vi "mqttInterpretSubscribtionData.vi"(0 "rxTelegram in":u8[](array[numeric]) format="%02x", 5 "qos":T1, 11 "error in (no error)":errorcluster) -> (4 "topic":string, 6 "value":string, 8 "messageID":u16, 15 "error out":errorcluster)   [LabVIEW 2015, in "mqtt.lvclass"]
uses:
  mqtt.lvclass
  mqttTypedef/mqttQOSlevel.ctl
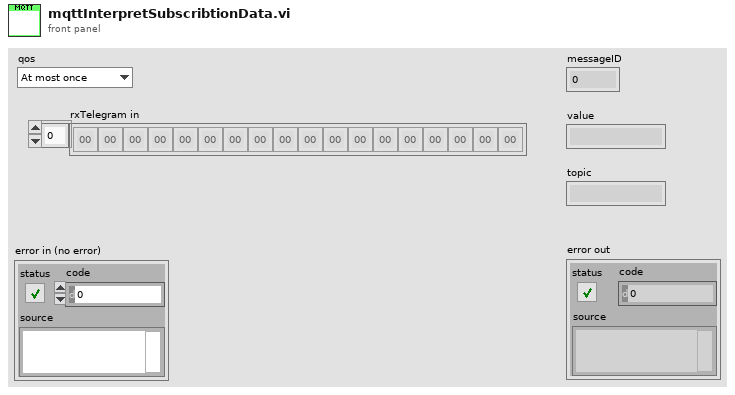
[diagram p1: front panel]
types:
  T1 = typedef "mqttQOSlevel.ctl" = enum8{"At most once", "At least once", "Exactly once", "Reserved"}
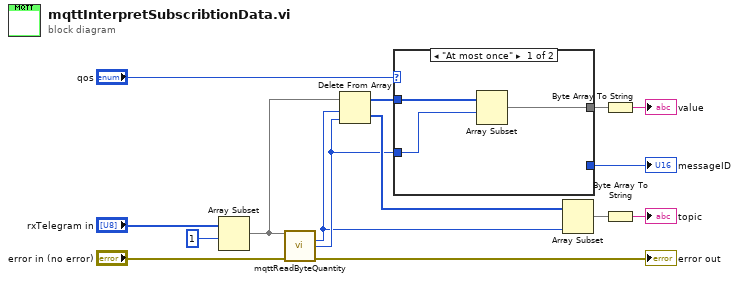
[diagram p0: block diagram]
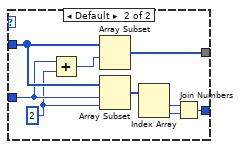
[diagram p2: hidden frame]
diagram:
  n1 = Array Subset(array="rxTelegram in", index=1) -> (w6:u8[])  [unwired: 1 in]
  n2 = call "mqttReadByteQuantity.vi"("rxTelegram in"=w6, "error in (no error)"="error in (no error)") -> ("remainingLength"=w1:i32, "lengthByteQuantity"=w2:i32, "error out"=→"error out":errorcluster)  [unwired: 11 in]
  n3 = Delete From Array(array=w6, length=w1, index=w2) -> (deleted portion=w4:u8[], array with subset deleted=w3:u8[])
  n4 = case shown="\"At most once\"" "qos" {
    tunnel: w3 -> [w18 w22]
    tunnel: [_ w25] -> w12
    tunnel: [w17 w23] -> w5
    tunnel: w2 -> [w16 w21]
    frame "At most once" {
      n5 = Array Subset(array=w18, index=w16) -> (w17:u8[])  [unwired: 1 in]
    }
    frame Default {
      w20 = 2 ("length")
      n6 = Add(x=w21, y=w20) -> (x+y=w19:i32)
      n7 = Array Subset(array=w22, index=w19) -> (w23:u8[])  [unwired: 1 in]
      n8 = Array Subset(array=w22, index=w21, length=w20) -> (w24:u8[])
      n9 = Index Array(array=w24) -> (element #1=w27:u8, element #2=w26:u8)  [unwired: 2 in]
      n10 = Join Numbers(hi=w27, lo=w26) -> ((hi.lo)=w25:u16)
    }
  }
  "messageID" <- w12
  n11 = Array Subset(array=w4, length=w1) -> (w8:u8[])  [unwired: 1 in]
  n12 = Byte Array To String(unsigned byte array=w5) -> (string=→"value":string)
  n13 = Byte Array To String(unsigned byte array=w8) -> (string=→"topic":string)
